vi "RELAYS Read the Dev Addr.vi"(8 "error in (no error)":errorcluster, 11 "VISA resource name":refnum<visa-resource-name>) -> (0 "error out":errorcluster, 1 "Dev Address":u8, 2 "ack":string, 3 "VISA resource name out":refnum<visa-resource-name>)   [LabVIEW 2016, in "MB _relays.lvlib"]
uses:
  MB _relays.lvlib
  private/gen MB frame -read device address.vi
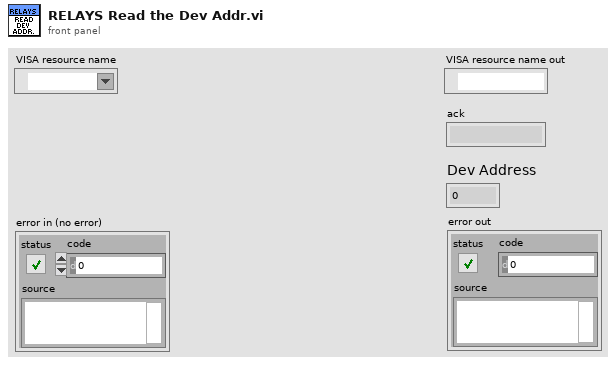
[diagram p1: front panel]
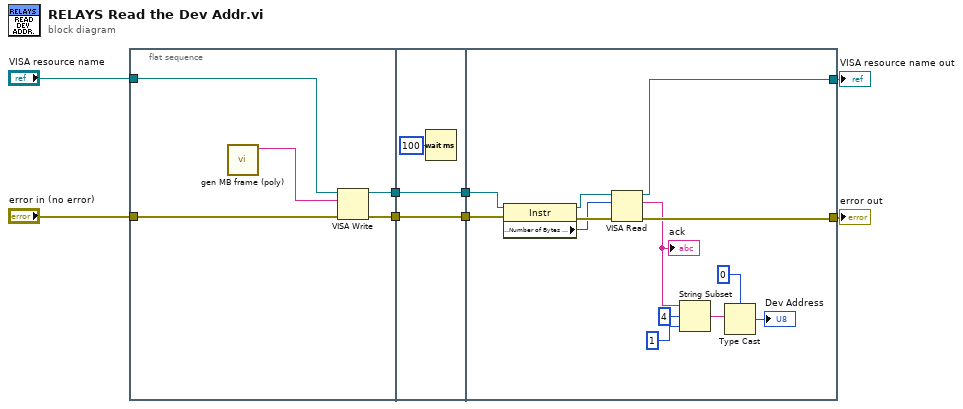
[diagram p0: block diagram]
diagram:
  n1 = flat-sequence {
    tunnel: "error in (no error)" -> [w10]
    tunnel: "VISA resource name" -> [w9]
    tunnel: [w13] -> w4
    tunnel: [w12] -> w3
    tunnel: w4 -> [w16]
    tunnel: w3 -> [w15]
    tunnel: [w16] -> w2
    tunnel: [w15] -> w1
    tunnel: [w23] -> w7
    tunnel: [w24] -> w8
    tunnel: w2 -> [w28]
    tunnel: w1 -> [w29]
    frame #0 {
      n2 = call-poly "gen MB frame (poly).vi"() -> ("MB frame"=w11:string)  [unwired: 11 in]
      n3 = VISA Write(VISA resource name=w9, write buffer=w11, error in (no error)=w10) -> (VISA resource name out=w13:refnum<visa-resource-name>, error out=w12:errorcluster)  [unwired: 1 out]
    }
    frame #1 {
      n4 = Wait (ms)(milliseconds to wait=u32 100) -> ()  [unwired: 1 out]
    }
    frame #2 {
      n5 = property class="Instr"(reference=w28, error in=w29) -> (reference out=w26:refnum<visa-resource-name>, error out=w27:errorcluster, "Serial Settings:Number of Bytes at Serial Port"=w25:u32)
      n6 = VISA Read(VISA resource name=w26, byte count=w25, error in (no error)=w27) -> (VISA resource name out=w24:refnum<visa-resource-name>, read buffer=w22:string, error out=w23:errorcluster)  [unwired: 1 out]
      "ack" <- w22
      n7 = String Subset(string=w22, offset (0)=4, length (rest)=1 ("length (rest)")) -> (substring=w19:string)
      n8 = Type Cast(type=u8 0, x=w19) -> (*(type *) &x=→"Dev Address":u8)
    }
  }
  "VISA resource name out" <- w8
  "error out" <- w7
